vi "mod_toolkit_example.vi"() -> ()   [LabVIEW 2011]
doc: "Modulation Toolkit Example for RTL-SDR"
uses:
  <vilib>/measure/maresamp.llb/Resample Waveform (continuous).vi
  <vilib>/Waveform/WDTOps.llb/WDT Append Waveforms DBL.vi
  <vilib>/addons/Modulation/niAMT.lvlib
  <vilib>/measure/NI_MAPro.lvlib
panel:
  out "Bytes processed":i32
  in  "Boolean":bool
  out "error out":errorcluster
  in  "LO frequency":i32=100000000
  in  "address":string="127.0.0.1"
  in  "remote port":u16=1234
  # "How to use:"
  # "This VI can be used to demodulate and listen to FM broadcast transmissions."
  # "Step #1: Start rtl_tcp (you might do it with START_RTL_TCP.bat) and enter parameters here."
  # "Step #2: Enter your favourite FM radio station's frequency in Herz."
  # "Step #3: Run the VI."
  # "Step #3: Press the \"Stop recording\" button after a few seconds."
  # "Step #4: Listen to the demodulated audio."
  # "Good luck and have fun!      Andris, HA7ILM"
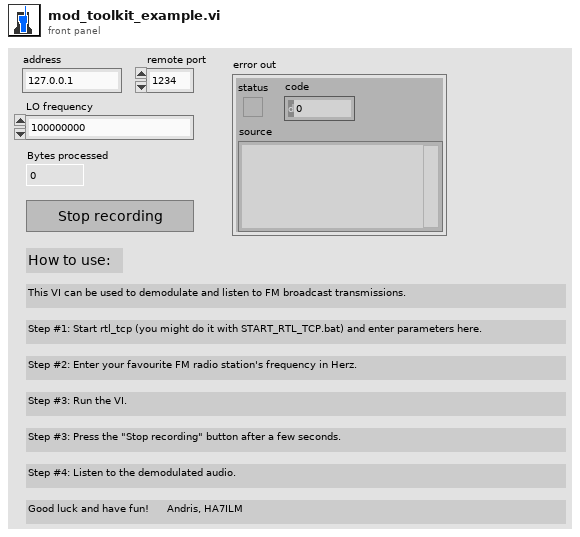
[diagram p1: front panel]
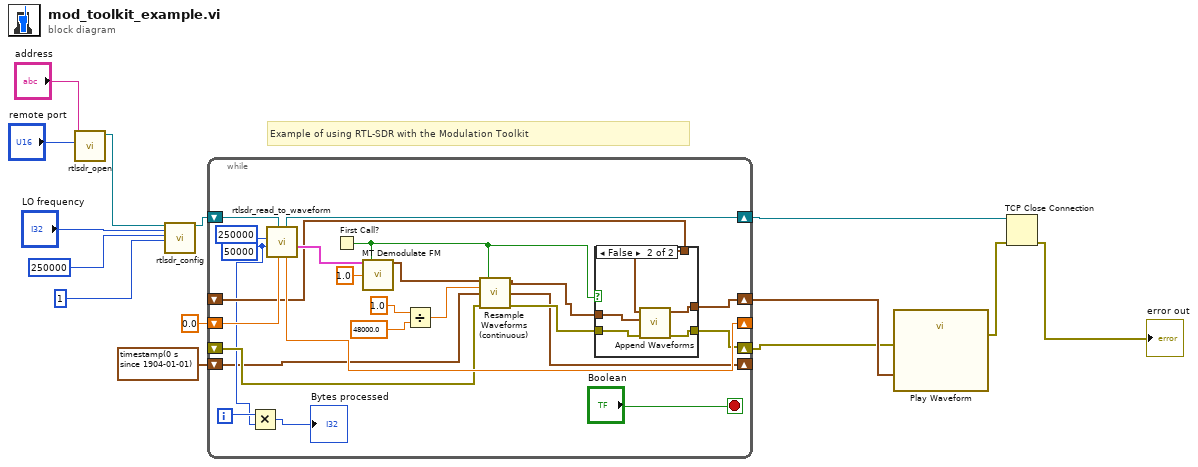
[diagram p0: block diagram]
diagram:
  # "Example of using RTL-SDR with the Modulation Toolkit"
  n1 = call "rtlsdr_open.vi"("remote port"="remote port", "address"="address") -> ("ref"=w12:refnum<k5>)  [unwired: 8 in, 1 out]
  n2 = call "rtlsdr_config.vi"("ref in"=w12, "LO frequency"="LO frequency", "Samplerate"=250000, "Autogain"=1) -> ("ref out"=w8:refnum<k5>)  [unwired: 14 in, 1 out]
  n3 = while {
    shift-right: [w34] -> w3
    shift-left: w8 -> [w38]
    shift-right: [w32] -> _
    shift-left: 0.0 ("next timestamp index") -> [w33]
    shift-right: [w28] -> w6
    shift-left: _ -> [w27]
    shift-right: [w24] -> w5
    shift-left: _ -> [w23]
    shift-right: [w16] -> _
    shift-left: timestamp(0 s since 1904-01-01) ("next t0") -> [w17]
    i -> [w20]
    stop <- "Boolean" stop-if-true
    w19 = 50000 ("buffer size")
    n4 = Multiply(x=w20, y=w19) -> (x*y=→"Bytes processed":i32)
    n5 = call "rtlsdr_read_to_waveform.vi"("timestamp index"=w33, "ref in"=w38, "buffer size"=w19, "sample rate"=250000) -> ("output downconverted waveform"=w30:cluster{dbl, dbl, cdb[]}, "next timestamp index"=w32:dbl, "ref out"=w34:refnum<k5>)  [unwired: 2 in, 3 out]
    n6 = First Call?() -> (First Call?: T/F=w22:bool)
    n7 = call <vilib>:"MT Demodulate FM.vi"("FM modulated waveform"=w30, "reset? (F)"=w22, "FM deviation (Hz)"=1.0) -> ("FM demodulated waveform"=w29:waveform(dbl))  [unwired: 10 in, 2 out]
    n8 = Divide(x=1.0 ("dt"), y=48000.0 ("dt")) -> (x/y=w35:dbl)
    n9 = call-poly <vilib>:"Resample Waveforms (continuous).vi"("waveform in"=w29, "reset"=w22, "dt"=w35, "t0"=w17, "error in (no error)"=w23) -> ("resampled waveform out"=w26:waveform(dbl), "next t0"=w16:timestamp, "error out"=w25:errorcluster)  [unwired: 6 in, 2 out]
    n10 = case shown="False" w22 {
      tunnel: [w40 w45] -> w28
      tunnel: w27 -> [_ w44]
      tunnel: w26 -> [w40 w43]
      tunnel: w25 -> [w39 w42]
      tunnel: [w39 w41] -> w24
      frame True {
      }
      frame False {
        n11 = call-poly <vilib>:"Append Waveforms.vi"("error in (no error)"=w42, "waveform B"=w43, "waveform A"=w44) -> ("error out"=w41:errorcluster, "waveform out"=w45:waveform(dbl))  [unwired: 7 in]
      }
    }
  }
  n12 = call "Play Waveform"("Data"=w6, "error in"=w5) -> ("error out"=w2:errorcluster)  [unwired: 17 in]
  n13 = TCP Close Connection(connection ID=w3, error in (no error)=w2) -> (error out=→"error out":errorcluster)  [unwired: 1 in, 1 out]
